vi "Printable variable.vi"(8 "error in (no error)":errorcluster caption="entrée d'erreur (pas d'erreur)", 11 "Function":enum16{"Get Variables", "Reset"}(ring)) -> (0 "error out":errorcluster caption="sortie d'erreur", 3 "Printable Variable":string[](array[string]))   [LabVIEW 2020]
uses:
  TypeDef/Variable Printable.ctl
  Library Commun.lvlib
panel:
  in  "Variable Printable":T1
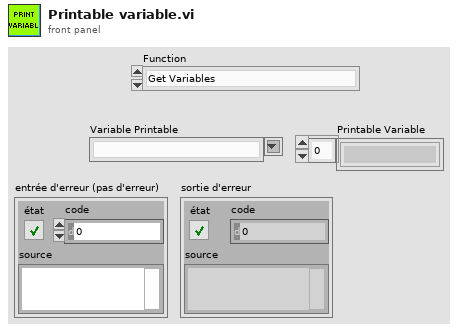
[diagram p1: front panel]
types:
  T1 = typedef "Variable Printable.ctl" = string
  T2 = enum16{"Get Variable", "Get All Variables", "Set Variable", "Delete Variable", "Delete All Variable"}
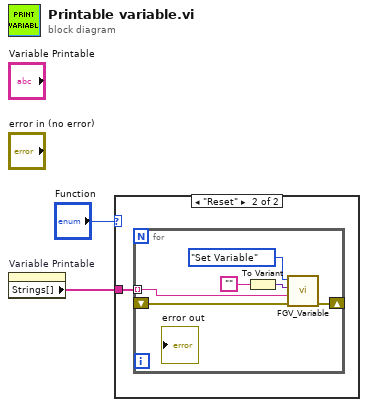
[diagram p0: block diagram]
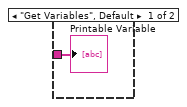
[diagram p2: hidden frame]
diagram:
  n1 = property on="Variable Printable" class="ChneDér (strict)"() -> ("Strings[]"=w1:string[])  [unwired: 2 in, 2 out]
  n2 = case shown="\"Reset\"" "Function" {
    tunnel: w1 -> [w3 w4]
    frame "Get Variables", Default {
      "Printable Variable" <- w3
    }
    frame "Reset" {
      n3 = for {
        shift-right: [w6] -> _
        shift-left: _ -> [w9]
        tunnel: w4 -> [w5] mode=indexing
        n4 = To Variant(anything="") -> (Variant=w8:variant)
        n5 = call "FGV_Variable.vi"("error in (no error)"=w9, "Variable"=w5, "Data In"=w8, "Function"=T2."Set Variable") -> ("error out"=w6:errorcluster)  [unwired: 5 in, 2 out]
      }
    }
  }
